vi "SP_OEE_2_test.vi"() -> ()   [LabVIEW 2017] (continued)
                      tunnel: w14784 -> [w15083]
                      tunnel: w14783 -> [w15091]
                      tunnel: w14782 -> [w15081]
                      tunnel: w14781 -> [w15090]
                      tunnel: w14780 -> [w15079]
                      tunnel: w14779 -> [w15089]
                      tunnel: w14778 -> [w15077]
                      tunnel: w14777 -> [w15113]
                      tunnel: w14776 -> [w15112]
                      tunnel: w14775 -> [w15088]
                      tunnel: w14774 -> [w15075]
                      tunnel: [w15113] -> w14772
                      tunnel: [w15112] -> w14771
                      tunnel: [w15106] -> w14770
                      tunnel: [w15099] -> w14769
                      tunnel: [w15098] -> w14768
                      tunnel: [w15097] -> w14767
                      tunnel: [w15096] -> w14766
                      tunnel: [w15095] -> w14765
                      tunnel: [w15094] -> w14764
                      tunnel: [w15093] -> w14763
                      tunnel: [w15092] -> w14762
                      tunnel: [w15091] -> w14761
                      tunnel: [w15090] -> w14760
                      tunnel: [w15089] -> w14759
                      tunnel: [w15088] -> w14758
                      tunnel: [w15073] -> w14757
                      tunnel: w14773 -> [w15073]
                      tunnel: [w15126] -> _
                      tunnel: [w15122] -> _
                      tunnel: w14772 -> [w15123]
                      tunnel: w14771 -> [w15126]
                      tunnel: w14770 -> [w15117]
                      tunnel: w14769 -> [w15124]
                      tunnel: w14768 -> [_]
                      tunnel: w14767 -> [_]
                      tunnel: w14766 -> [w15116]
                      tunnel: w14765 -> [_]
                      tunnel: w14764 -> [_]
                      tunnel: w14763 -> [w15118]
                      tunnel: w14762 -> [_]
                      tunnel: w14761 -> [_]
                      tunnel: w14760 -> [w15114]
                      tunnel: w14759 -> [_]
                      tunnel: w14758 -> [_]
                      tunnel: w14757 -> [w15121]
                      frame #0 {
                        w14861 = "%Y-%m-%d" ("time format string (%c)")
                        n2698 = Decimal String To Number(string=w14847) -> (number=w14848:i32)  [unwired: 2 in, 1 out]
                        n2699 = property on="Table" class="Tbl (strict)"("Visible"=TRUE) -> ()  [unwired: 2 in, 2 out]
                        n2700 = Format Date/Time String(time format string (%c)=w14861, seconds (now)=w14853) -> (date/time string=w14862:string)  [unwired: 1 in]
                        n2701 = Format Date/Time String(time format string (%c)=w14861, seconds (now)=w14852) -> (date/time string=w14860:string)  [unwired: 1 in]
                        n2702 = Format Into String(format string="Where BREAKDOWN_DATE between '%s' and '%s' and  SHIFT_ID = '%d'  ", w14862, w14860, w14848) -> (resulting string=w14859:string)  [unwired: 2 in, 1 out]
                        n2703 = call <vilib>:"DB Tools Select Data.vi"("condition"=w14859, "error in (no error)"=w14868, "columns"=string[] ["BREAKDOWN_DATE"], "table"="STATION_1_LOG_HISTORY", "connection reference"=w14870) -> ("error out"=w14855:errorcluster, "data"=w14858:variant[][], "connection reference out"=w14869:T2)  [unwired: 1 in]
                        n2704 = property on="Table 2" class="Tbl (strict)"("Visible"=FALSE) -> ()  [unwired: 2 in, 2 out]
                        n2705 = xnode "Database Variant To Data"("database variant"=w14858, "error in (no error)"=w14855, "type"=string[][] [] ("Elements Found")) -> ("data"=w14856:string[][], "error out"=w14854:errorcluster)
                        n2706 = Index Array(array=w14856, index (col)=0 ("disabled index (col)")) -> (element=w14864:string[])  [unwired: 1 in]
                        n2707 = call "Search_1d_array_element.vi"("Count in"=string[] [] ("Elements Found"), "BD Date"=w14864, "Elements Found in"=string[] [] ("Elements Found")) -> ("Elements Found out"=w14851:string[])  [unwired: 4 in, 2 out]
                        n2708 = Build Array(w14851) -> (w14874:string[][])
                        n2709 = Transpose 2D Array(2D array=w14874) -> (transposed array=w14873:string[][])
                      }
                      frame #1 {
                        n2710 = disable-structure shown="Enabled" {
                          disable-tunnel: w14936 -> [w14947 w14949]
                          disable-tunnel: [w14946 w14949] -> w14935
                          disable-tunnel: w14934 -> [w14945 w14950]
                          disable-tunnel: [w14944 w14950] -> w14933
                          disable-tunnel: w14931 -> [w14942 _]
                          disable-tunnel: w14930 -> [w14941 _]
                          disable-tunnel: [w14940 _] -> w14929
                          disable-tunnel: [w14939 _] -> w14926
                          disable-tunnel: w14924 -> [w14938 _]
                          disable-tunnel: w14921 -> [w14937 w14948]
                          disable-tunnel: [_ w14948] -> w14920
                          frame Disabled {
                            n2711 = call "Stack_holderwise_total_bd_count_&_duration_2.vi"("Refnum in"=w14947, "BREAKDOWN_STK_HOLD_ID"=1, "condition"=w14938, "Form Date"=w14942, "To Date"=w14941, "error in (no error)"=w14945, "Shift"=w14937) -> ("Refnum out"=w14946:T2, "Count out"=w14940:string[], "appended array"=w14939:dbl[], "error out"=w14944:errorcluster)  [unwired: 5 in]
                          }
                          frame Enabled {
                          }
                        }
                        n2712 = call "NUMERIC TO STRING.vi"("appended array"=w14926) -> ("Array"=w14925:string[])  [unwired: 4 in]
                        n2713 = call "Insert_empty_element_with_zero.vi"("searched date"=w14929, "fixed date"=w14927) -> ("O/P"=w14922:string[])  [unwired: 9 in]
                        n2714 = call "Insert_empty_element_with_zero.vi"("searched date"=w14925, "fixed date"=w14927) -> ("O/P"=w14928:string[])  [unwired: 9 in]
                      }
                      frame #2 {
                        n2715 = disable-structure shown="Enabled" {
                          disable-tunnel: w14966 -> [w14980 w14982]
                          disable-tunnel: [w14979 w14982] -> w14965
                          disable-tunnel: w14964 -> [w14978 w14983]
                          disable-tunnel: [w14977 w14983] -> w14963
                          disable-tunnel: w14962 -> [w14976 _]
                          disable-tunnel: w14961 -> [w14975 _]
                          disable-tunnel: [w14974 _] -> w14960
                          disable-tunnel: [w14973 _] -> w14956
                          disable-tunnel: w14954 -> [w14972 _]
                          disable-tunnel: w14952 -> [w14970 w14981]
                          disable-tunnel: [_ w14981] -> w14951
                          frame Disabled {
                            n2716 = call "Stack_holderwise_total_bd_count_&_duration_2.vi"("Refnum in"=w14978, "BREAKDOWN_STK_HOLD_ID"=2, "condition"=w14972, "Form Date"=w14976, "To Date"=w14975, "error in (no error)"=w14980, "Shift"=w14970) -> ("Refnum out"=w14977:T2, "Count out"=w14974:string[], "appended array"=w14973:dbl[], "error out"=w14979:errorcluster)  [unwired: 5 in]
                          }
                          frame Enabled {
                          }
                        }
                        n2717 = call "Insert_empty_element_with_zero.vi"("searched date"=w14960, "fixed date"=w14957) -> ("O/P"=w14959:string[])  [unwired: 9 in]
                        n2718 = call "NUMERIC TO STRING.vi"("appended array"=w14956) -> ("Array"=w14955:string[])  [unwired: 4 in]
                        n2719 = call "Insert_empty_element_with_zero.vi"("searched date"=w14955, "fixed date"=w14957) -> ("O/P"=w14958:string[])  [unwired: 9 in]
                      }
                      frame #3 {
                        n2720 = call "Stack_holderwise_total_bd_count_&_duration_2.vi"("Refnum in"=w14997, "BREAKDOWN_STK_HOLD_ID"=3, "condition"=w14987, "Form Date"=w14995, "To Date"=w14994, "error in (no error)"=w14999, "Shift"=w14984) -> ("Refnum out"=w14996:T2, "Count out"=w14993:string[], "appended array"=w14989:dbl[], "error out"=w14998:errorcluster)  [unwired: 5 in]
                        n2721 = call "Insert_empty_element_with_zero.vi"("searched date"=w14993, "fixed date"=w14990) -> ("O/P"=w14992:string[])  [unwired: 9 in]
                        n2722 = call "NUMERIC TO STRING.vi"("appended array"=w14989) -> ("Array"=w14988:string[])  [unwired: 4 in]
                        n2723 = call "Insert_empty_element_with_zero.vi"("searched date"=w14988, "fixed date"=w14990) -> ("O/P"=w14991:string[])  [unwired: 9 in]
                      }
                      frame #4 {
                        n2724 = disable-structure shown="Enabled" {
                          disable-tunnel: w15018 -> [w15034 w15037]
                          disable-tunnel: w15017 -> [w15033 w15036]
                          disable-tunnel: [w15032 w15036] -> w15016
                          disable-tunnel: [w15031 w15037] -> w15015
                          disable-tunnel: w15014 -> [w15030 _]
                          disable-tunnel: w15013 -> [w15029 _]
                          disable-tunnel: [w15028 _] -> w15012
                          disable-tunnel: [w15027 _] -> w15008
                          disable-tunnel: w15006 -> [w15026 _]
                          frame Disabled {
                            n2725 = call "Stack_holderwise_total_bd_count_&_duration.vi"("Refnum in"=w15033, "BREAKDOWN_STK_HOLD_ID"=4, "condition"=w15026, "Form Date"=w15030, "To Date"=w15029, "error in (no error)"=w15034) -> ("Refnum out"=w15032:T2, "Count out"=w15028:string[], "appended array"=w15027:dbl[], "error out"=w15031:errorcluster)  [unwired: 6 in]
                          }
                          frame Enabled {
                          }
                        }
                        n2726 = call "Insert_empty_element_with_zero.vi"("searched date"=w15012, "fixed date"=w15009) -> ("O/P"=w15011:string[])  [unwired: 9 in]
                        n2727 = call "NUMERIC TO STRING.vi"("appended array"=w15008) -> ("Array"=w15007:string[])  [unwired: 4 in]
                        n2728 = call "Insert_empty_element_with_zero.vi"("searched date"=w15007, "fixed date"=w15009) -> ("O/P"=w15010:string[])  [unwired: 9 in]
                      }
                      frame #5 {
                        n2729 = disable-structure shown="Enabled" {
                          disable-tunnel: w15051 -> [w15069 w15072]
                          disable-tunnel: [w15068 w15072] -> w15050
                          disable-tunnel: w15049 -> [w15067 w15071]
                          disable-tunnel: [w15066 w15071] -> w15048
                          disable-tunnel: w15047 -> [w15065 _]
                          disable-tunnel: w15046 -> [w15064 _]
                          disable-tunnel: [w15063 _] -> w15045
                          disable-tunnel: [w15062 _] -> w15041
                          disable-tunnel: w15039 -> [w15061 _]
                          frame Disabled {
                            n2730 = call "Stack_holderwise_total_bd_count_&_duration.vi"("Refnum in"=w15067, "BREAKDOWN_STK_HOLD_ID"=5, "condition"=w15061, "Form Date"=w15064, "To Date"=w15065, "error in (no error)"=w15069) -> ("Refnum out"=w15066:T2, "Count out"=w15063:string[], "appended array"=w15062:dbl[], "error out"=w15068:errorcluster)  [unwired: 6 in]
                          }
                          frame Enabled {
                          }
                        }
                        n2731 = call "NUMERIC TO STRING.vi"("appended array"=w15041) -> ("Array"=w15040:string[])  [unwired: 4 in]
                        n2732 = call "Insert_empty_element_with_zero.vi"("searched date"=w15045, "fixed date"=w15043) -> ("O/P"=w15044:string[])  [unwired: 9 in]
                        n2733 = call "Insert_empty_element_with_zero.vi"("searched date"=w15040, "fixed date"=w15043) -> ("O/P"=w15042:string[])  [unwired: 9 in]
                      }
                      frame #6 {
                        n2734 = call "String to numeric.vi"("Array"=w15083) -> ("Array 2"=w15082:dbl[])  [unwired: 4 in]
                        n2735 = call "String to numeric.vi"("Array"=w15081) -> ("Array 2"=w15080:dbl[])  [unwired: 4 in]
                        n2736 = call "String to numeric.vi"("Array"=w15079) -> ("Array 2"=w15078:dbl[])  [unwired: 4 in]
                        n2737 = call "String to numeric.vi"("Array"=w15077) -> ("Array 2"=w15076:dbl[])  [unwired: 4 in]
                        n2738 = call "String to numeric.vi"("Array"=w15075) -> ("Array 2"=w15074:dbl[])  [unwired: 4 in]
                        n2739 = Decimal String To Number(string=w15088) -> (number=w15107:i32[])  [unwired: 2 in, 1 out]
                        n2740 = Decimal String To Number(string=w15089) -> (number=w15108:i32[])  [unwired: 2 in, 1 out]
                        n2741 = Decimal String To Number(string=w15090) -> (number=w15109:i32[])  [unwired: 2 in, 1 out]
                        n2742 = Decimal String To Number(string=w15091) -> (number=w15110:i32[])  [unwired: 2 in, 1 out]
                        n2743 = Decimal String To Number(string=w15092) -> (number=w15105:i32[])  [unwired: 2 in, 1 out]
                        n2744 = Compound Arithmetic op=ADD(w15082, w15080, w15078, w15076, w15074) -> (w15085:dbl[])
                        n2745 = Build Array(w15083) -> (w15104:string[][])
                        n2746 = Build Array(w15081) -> (w15103:string[][])
                        n2747 = Build Array(w15079) -> (w15102:string[][])
                        n2748 = Build Array(w15077) -> (w15101:string[][])
                        n2749 = Build Array(w15075) -> (w15100:string[][])
                        n2750 = Number To Fractional String(number=w15085, precision (6)=i16 2) -> (F-format string=w15084:string[])  [unwired: 2 in]
                        n2751 = Compound Arithmetic op=ADD(w15107, w15108, w15109, w15110, w15105) -> (w15111:i32[])
                        n2752 = Transpose 2D Array(2D array=w15104) -> (transposed array=w15098:string[][])
                        n2753 = Transpose 2D Array(2D array=w15103) -> (transposed array=w15097:string[][])
                        n2754 = Transpose 2D Array(2D array=w15102) -> (transposed array=w15096:string[][])
                        n2755 = Transpose 2D Array(2D array=w15101) -> (transposed array=w15095:string[][])
                        n2756 = Transpose 2D Array(2D array=w15100) -> (transposed array=w15094:string[][])
                        n2757 = Number To Decimal String(number=w15111) -> (decimal integer string=w15106:string[])  [unwired: 1 in]
                        n2758 = Build Array(w15084) -> (w15087:string[][])
                        n2759 = Transpose 2D Array(2D array=w15087) -> (transposed array=w15093:string[][])
                      }
                      frame #7 {
                        w15115 = string[] [""]
                        n2760 = Insert Into Array(array=w15124, index (col)=1 ("disabled index (col)"), new element #1=w15115, new element #2=w15115, new element #3=w15115, new element #4=w15115, new element #5=w15114, new element #6=w15116, new element #7=w15115, new element #8=w15115, new element #9=w15115, new element #10=w15115, new element #11=w15117, new element #12=w15118) -> (w15120:string[][])  [unwired: 1 in]
                        n2761 = call "flot graph for month n year.vi"("BD Date"=w15121, "error in (no error)"=w15123, "Count total"=w15117) -> ("error out"=w15122:errorcluster, "Run-Time Status"=w15119:cluster{"Array 2":timestamp[], dbl[]})  [unwired: 7 in]
                        n2762 = local write "Run-Time Status"(w15119) -> ()
                        n2763 = local write "Table"(w15120) -> ()
                      }
                    }
                  }
                  frame "all" {
                  }
                }
              }
              frame "Quality" {
                n2764 = local read "Shift"() -> (w15127:string)
                n2765 = case shown="\"3\"" w15127 {
                  selector: w15127 -> [_ w15501 w15885 w16269 _]
                  tunnel: w15132 -> [w15137 w15506 w15890 w16274 _]
                  tunnel: w15131 -> [w15136 w15505 w15889 w16273 _]
                  tunnel: w15130 -> [w15135 w15504 w15888 w16272 _]
                  tunnel: w15129 -> [w15134 w15503 w15887 w16271 _]
                  tunnel: w15128 -> [w15133 w15502 w15886 w16270 _]
                  frame "ALL", Default {
                    n2766 = flat-sequence {
                      tunnel: w15137 -> [w15249]
                      tunnel: w15136 -> [w15247]
                      tunnel: [w15233] -> w15227
                      tunnel: [w15248] -> w15226
                      tunnel: w15135 -> [_]
                      tunnel: [w15252] -> w15225
                      tunnel: [w15232] -> w15224
                      tunnel: [w15231] -> w15223
                      tunnel: [w15229] -> w15222
                      tunnel: w15134 -> [w15232]
                      tunnel: w15133 -> [w15231]
                      tunnel: ["Where BREAKDOWN_DATE between '%s'and '%s' and BREAKDOWN_STK_HOLD_ID ='%d'  "] -> w15221
                      tunnel: [w15229] -> w15220
                      tunnel: w15227 -> [w15311]
                      tunnel: w15226 -> [w15313]
                      tunnel: w15225 -> [w15309]
                      tunnel: w15224 -> [w15308]
                      tunnel: w15223 -> [w15307]
                      tunnel: [w15310] -> w15219
                      tunnel: [w15312] -> w15218
                      tunnel: [w15309] -> w15217
                      tunnel: [w15299] -> w15216
                      tunnel: [w15305] -> w15215
                      tunnel: [w15308] -> w15214
                      tunnel: [w15307] -> w15213
                      tunnel: w15222 -> [w15304]
                      tunnel: [w15304] -> w15212
                      tunnel: w15221 -> [w15301]
                      tunnel: [w15301] -> w15211
                      tunnel: [w15300] -> w15210
                      tunnel: w15220 -> [w15300]
                      tunnel: w15219 -> [w15339]
                      tunnel: w15218 -> [w15337]
                      tunnel: w15217 -> [w15342]
                      tunnel: w15216 -> [w15341]
                      tunnel: w15215 -> [w15340]
                      tunnel: w15214 -> [w15335]
                      tunnel: w15213 -> [w15334]
                      tunnel: [w15342] -> w15209
                      tunnel: [w15341] -> w15208
                      tunnel: [w15340] -> w15207
                      tunnel: [w15338] -> w15206
                      tunnel: [w15332] -> w15205
                      tunnel: [w15331] -> w15204
                      tunnel: [w15336] -> w15203
                      tunnel: [w15335] -> w15202
                      tunnel: [w15334] -> w15201
                      tunnel: w15212 -> [w15330]
                      tunnel: [w15330] -> w15200
                      tunnel: w15211 -> [w15327]
                      tunnel: [w15327] -> w15199
                      tunnel: [w15326] -> w15198
                      tunnel: w15210 -> [w15326]
                      tunnel: w15209 -> [w15373]
                      tunnel: w15208 -> [w15372]
                      tunnel: w15207 -> [w15371]
                      tunnel: w15206 -> [w15368]
                      tunnel: w15205 -> [w15370]
                      tunnel: w15204 -> [w15369]
                      tunnel: w15203 -> [w15366]
                      tunnel: w15202 -> [w15364]
                      tunnel: w15201 -> [w15363]
                      tunnel: [w15373] -> w15197
                      tunnel: [w15372] -> w15196
                      tunnel: [w15371] -> w15195
                      tunnel: [w15370] -> w15194
                      tunnel: [w15369] -> w15193
                      tunnel: [w15367] -> w15192
                      tunnel: [w15361] -> w15191
                      tunnel: [w15360] -> w15190
                      tunnel: [w15365] -> w15189
                      tunnel: [w15364] -> w15188
                      tunnel: [w15363] -> w15187
                      tunnel: w15200 -> [w15359]
                      tunnel: [w15359] -> w15186
                      tunnel: w15199 -> [w15356]
                      tunnel: [w15356] -> w15185
                      tunnel: [w15355] -> w15184
                      tunnel: w15198 -> [w15355]
                      tunnel: w15197 -> [w15407]
                      tunnel: w15196 -> [w15406]
                      tunnel: w15195 -> [w15405]
                      tunnel: w15194 -> [w15404]
                      tunnel: w15193 -> [w15403]
                      tunnel: w15192 -> [w15400]
                      tunnel: w15191 -> [w15402]
                      tunnel: w15190 -> [w15401]
                      tunnel: w15189 -> [w15399]
                      tunnel: w15188 -> [w15396]
                      tunnel: w15187 -> [w15395]
                      tunnel: [w15407] -> w15183
                      tunnel: [w15406] -> w15182
                      tunnel: [w15405] -> w15181
                      tunnel: [w15404] -> w15180
                      tunnel: [w15403] -> w15179
                      tunnel: [w15402] -> w15178
                      tunnel: [w15401] -> w15177
                      tunnel: [w15398] -> w15176
                      tunnel: [w15397] -> w15175
                      tunnel: [w15393] -> w15174
                      tunnel: [w15392] -> w15173
                      tunnel: [w15396] -> w15172
                      tunnel: [w15395] -> w15171
                      tunnel: w15186 -> [w15391]
                      tunnel: [w15391] -> w15170
                      tunnel: w15185 -> [w15388]
                      tunnel: [w15388] -> w15169
                      tunnel: [w15387] -> w15168
                      tunnel: w15184 -> [w15387]
                      tunnel: w15183 -> [w15430]
                      tunnel: w15182 -> [w15429]
                      tunnel: w15181 -> [w15428]
                      tunnel: w15180 -> [w15427]
                      tunnel: w15179 -> [w15426]
                      tunnel: w15178 -> [w15425]
                      tunnel: w15177 -> [w15424]
                      tunnel: w15176 -> [w15419]
                      tunnel: w15175 -> [w15421]
                      tunnel: w15174 -> [w15423]
                      tunnel: w15173 -> [w15422]
                      tunnel: w15172 -> [w15416]
                      tunnel: w15171 -> [w15417]
                      tunnel: [w15430] -> w15167
                      tunnel: [w15429] -> w15166
                      tunnel: [w15428] -> w15165
                      tunnel: [w15427] -> w15164
                      tunnel: [w15426] -> w15163
                      tunnel: [w15425] -> w15162
                      tunnel: [w15424] -> w15161
                      tunnel: [w15423] -> w15160
                      tunnel: [w15422] -> w15159
                      tunnel: [w15420] -> w15158
                      tunnel: [w15418] -> w15157
                      tunnel: [w15414] -> w15156
                      tunnel: [w15412] -> w15155
                      tunnel: w15170 -> [w15413]
                      tunnel: w15169 -> [w15409]
                      tunnel: [w15408] -> w15154
                      tunnel: w15168 -> [w15408]
                      tunnel: w15167 -> [w15469]
                      tunnel: w15166 -> [w15462]
                      tunnel: w15165 -> [w15453]
                      tunnel: w15164 -> [w15461]
                      tunnel: w15163 -> [w15451]
                      tunnel: w15162 -> [w15460]
                      tunnel: w15161 -> [w15449]
                      tunnel: w15160 -> [w15459]
                      tunnel: w15159 -> [w15447]
                      tunnel: w15158 -> [w15483]
                      tunnel: w15157 -> [w15482]
                      tunnel: w15156 -> [w15458]
                      tunnel: w15155 -> [w15445]
                      tunnel: [w15483] -> w15153
                      tunnel: [w15482] -> w15152
                      tunnel: [w15476] -> w15151
                      tunnel: [w15469] -> w15150
                      tunnel: [w15468] -> w15149
                      tunnel: [w15467] -> w15148
                      tunnel: [w15466] -> w15147
                      tunnel: [w15465] -> w15146
                      tunnel: [w15464] -> w15145
                      tunnel: [w15463] -> w15144
                      tunnel: [w15462] -> w15143
                      tunnel: [w15461] -> w15142
                      tunnel: [w15460] -> w15141
                      tunnel: [w15459] -> w15140
                      tunnel: [w15458] -> w15139
                      tunnel: [w15443] -> w15138
                      tunnel: w15154 -> [w15443]
                      tunnel: [w15496] -> _
                      tunnel: [w15492] -> _
                      tunnel: w15153 -> [w15493]
                      tunnel: w15152 -> [w15496]
                      tunnel: w15151 -> [w15487]
                      tunnel: w15150 -> [w15494]
                      tunnel: w15149 -> [_]
                      tunnel: w15148 -> [_]
                      tunnel: w15147 -> [_]
                      tunnel: w15146 -> [w15484]
                      tunnel: w15145 -> [_]
                      tunnel: w15144 -> [w15488]
                      tunnel: w15143 -> [_]
                      tunnel: w15142 -> [_]
                      tunnel: w15141 -> [_]
                      tunnel: w15140 -> [w15485]
                      tunnel: w15139 -> [_]
                      tunnel: w15138 -> [w15491]
                      frame #0 {
                        w15240 = "%Y-%m-%d" ("time format string (%c)")
                        n2767 = property on="Table" class="Tbl (strict)"("Visible"=TRUE) -> ()  [unwired: 2 in, 2 out]
                        n2768 = Format Date/Time String(time format string (%c)=w15240, seconds (now)=w15232) -> (date/time string=w15241:string)  [unwired: 1 in]
                        n2769 = Format Date/Time String(time format string (%c)=w15240, seconds (now)=w15231) -> (date/time string=w15239:string)  [unwired: 1 in]
                        n2770 = Format Into String(format string="Where BREAKDOWN_DATE between '%s' and '%s' ", w15241, w15239) -> (resulting string=w15238:string)  [unwired: 2 in, 1 out]
                        n2771 = call <vilib>:"DB Tools Select Data.vi"("condition"=w15238, "error in (no error)"=w15247, "columns"=string[] ["BREAKDOWN_DATE"], "table"="STATION_1_LOG_HISTORY", "connection reference"=w15249) -> ("error out"=w15234:errorcluster, "data"=w15237:variant[][], "connection reference out"=w15248:T2)  [unwired: 1 in]
                        n2772 = property on="Table 2" class="Tbl (strict)"("Visible"=FALSE) -> ()  [unwired: 2 in, 2 out]
                        n2773 = xnode "Database Variant To Data"("database variant"=w15237, "error in (no error)"=w15234, "type"=string[][] [] ("Elements Found")) -> ("data"=w15235:string[][], "error out"=w15233:errorcluster)
                        n2774 = Index Array(array=w15235, index (col)=0 ("disabled index (col)")) -> (element=w15243:string[])  [unwired: 1 in]
                        n2775 = call "Search_1d_array_element.vi"("Count in"=string[] [] ("Elements Found"), "BD Date"=w15243, "Elements Found in"=string[] [] ("Elements Found")) -> ("Elements Found out"=w15229:string[])  [unwired: 4 in, 2 out]
                        n2776 = Build Array(w15229) -> (w15253:string[][])
                        n2777 = Transpose 2D Array(2D array=w15253) -> (transposed array=w15252:string[][])
                      }
                      frame #1 {
                        n2778 = disable-structure shown="Enabled" {
                          disable-tunnel: w15313 -> [w15323 w15324]
                          disable-tunnel: [w15322 w15324] -> w15312
                          disable-tunnel: w15311 -> [w15321 w15325]
                          disable-tunnel: [w15320 w15325] -> w15310
                          disable-tunnel: w15308 -> [w15318 _]
                          disable-tunnel: w15307 -> [w15317 _]
                          disable-tunnel: [w15316 _] -> w15306
                          disable-tunnel: [w15315 _] -> w15303
                          disable-tunnel: w15301 -> [w15314 _]
                          frame Disabled {
                            n2779 = call "Stack_holderwise_total_bd_count_&_duration.vi"("Refnum in"=w15323, "BREAKDOWN_STK_HOLD_ID"=1, "condition"=w15314, "Form Date"=w15318, "To Date"=w15317, "error in (no error)"=w15321) -> ("Refnum out"=w15322:T2, "Count out"=w15316:string[], "appended array"=w15315:dbl[], "error out"=w15320:errorcluster)  [unwired: 6 in]
                          }
                          frame Enabled {
                          }
                        }
                        n2780 = call "NUMERIC TO STRING.vi"("appended array"=w15303) -> ("Array"=w15302:string[])  [unwired: 4 in]
                        n2781 = call "Insert_empty_element_with_zero.vi"("searched date"=w15306, "fixed date"=w15304) -> ("O/P"=w15299:string[])  [unwired: 9 in]
                        n2782 = call "Insert_empty_element_with_zero.vi"("searched date"=w15302, "fixed date"=w15304) -> ("O/P"=w15305:string[])  [unwired: 9 in]
                      }
                      frame #2 {
                        n2783 = disable-structure shown="Enabled" {
                          disable-tunnel: w15339 -> [w15352 w15354]
                          disable-tunnel: [w15351 w15354] -> w15338
                          disable-tunnel: w15337 -> [w15350 w15353]
                          disable-tunnel: [w15349 w15353] -> w15336
                          disable-tunnel: w15335 -> [w15348 _]
                          disable-tunnel: w15334 -> [w15347 _]
                          disable-tunnel: [w15346 _] -> w15333
                          disable-tunnel: [w15345 _] -> w15329
                          disable-tunnel: w15327 -> [w15344 _]
                          frame Disabled {
                            n2784 = call "Stack_holderwise_total_bd_count_&_duration.vi"("Refnum in"=w15350, "BREAKDOWN_STK_HOLD_ID"=2, "condition"=w15344, "Form Date"=w15348, "To Date"=w15347, "error in (no error)"=w15352) -> ("Refnum out"=w15349:T2, "Count out"=w15346:string[], "appended array"=w15345:dbl[], "error out"=w15351:errorcluster)  [unwired: 6 in]
                          }
                          frame Enabled {
                          }
                        }
                        n2785 = call "Insert_empty_element_with_zero.vi"("searched date"=w15333, "fixed date"=w15330) -> ("O/P"=w15332:string[])  [unwired: 9 in]
                        n2786 = call "NUMERIC TO STRING.vi"("appended array"=w15329) -> ("Array"=w15328:string[])  [unwired: 4 in]
                        n2787 = call "Insert_empty_element_with_zero.vi"("searched date"=w15328, "fixed date"=w15330) -> ("O/P"=w15331:string[])  [unwired: 9 in]
                      }
                      frame #3 {
                        n2788 = disable-structure shown="Enabled" {
                          disable-tunnel: w15368 -> [w15383 w15385]
                          disable-tunnel: [w15382 w15385] -> w15367
                          disable-tunnel: w15366 -> [w15381 w15384]
                          disable-tunnel: [w15380 w15384] -> w15365
                          disable-tunnel: w15364 -> [w15379 _]
                          disable-tunnel: w15363 -> [w15378 _]
                          disable-tunnel: [w15377 _] -> w15362
                          disable-tunnel: [w15376 _] -> w15358
                          disable-tunnel: w15356 -> [w15375 _]
                          frame Disabled {
                            n2789 = call "Stack_holderwise_total_bd_count_&_duration.vi"("Refnum in"=w15381, "BREAKDOWN_STK_HOLD_ID"=3, "condition"=w15375, "Form Date"=w15379, "To Date"=w15378, "error in (no error)"=w15383) -> ("Refnum out"=w15380:T2, "Count out"=w15377:string[], "appended array"=w15376:dbl[], "error out"=w15382:errorcluster)  [unwired: 6 in]
                          }
                          frame Enabled {
                          }
                        }
                        n2790 = call "Insert_empty_element_with_zero.vi"("searched date"=w15362, "fixed date"=w15359) -> ("O/P"=w15361:string[])  [unwired: 9 in]
                        n2791 = call "NUMERIC TO STRING.vi"("appended array"=w15358) -> ("Array"=w15357:string[])  [unwired: 4 in]
                        n2792 = call "Insert_empty_element_with_zero.vi"("searched date"=w15357, "fixed date"=w15359) -> ("O/P"=w15360:string[])  [unwired: 9 in]
                      }
                      frame #4 {
                        n2793 = call "Stack_holderwise_total_bd_count_&_duration.vi"("Refnum in"=w15399, "BREAKDOWN_STK_HOLD_ID"=4, "condition"=w15388, "Form Date"=w15396, "To Date"=w15395, "error in (no error)"=w15400) -> ("Refnum out"=w15398:T2, "Count out"=w15394:string[], "appended array"=w15390:dbl[], "error out"=w15397:errorcluster)  [unwired: 6 in]
                        n2794 = call "Insert_empty_element_with_zero.vi"("searched date"=w15394, "fixed date"=w15391) -> ("O/P"=w15393:string[])  [unwired: 9 in]
                        n2795 = call "NUMERIC TO STRING.vi"("appended array"=w15390) -> ("Array"=w15389:string[])  [unwired: 4 in]
                        n2796 = call "Insert_empty_element_with_zero.vi"("searched date"=w15389, "fixed date"=w15391) -> ("O/P"=w15392:string[])  [unwired: 9 in]
                      }
                      frame #5 {
                        n2797 = disable-structure shown="Enabled" {
                          disable-tunnel: w15421 -> [w15439 w15442]
                          disable-tunnel: [w15438 w15442] -> w15420
                          disable-tunnel: w15419 -> [w15437 w15441]
                          disable-tunnel: [w15436 w15441] -> w15418
                          disable-tunnel: w15417 -> [w15435 _]
                          disable-tunnel: w15416 -> [w15434 _]
                          disable-tunnel: [w15433 _] -> w15415
                          disable-tunnel: [w15432 _] -> w15411
                          disable-tunnel: w15409 -> [w15431 _]
                          frame Disabled {
                            n2798 = call "Stack_holderwise_total_bd_count_&_duration.vi"("Refnum in"=w15437, "BREAKDOWN_STK_HOLD_ID"=5, "condition"=w15431, "Form Date"=w15434, "To Date"=w15435, "error in (no error)"=w15439) -> ("Refnum out"=w15436:T2, "Count out"=w15433:string[], "appended array"=w15432:dbl[], "error out"=w15438:errorcluster)  [unwired: 6 in]
                          }
                          frame Enabled {
                          }
                        }
                        n2799 = call "NUMERIC TO STRING.vi"("appended array"=w15411) -> ("Array"=w15410:string[])  [unwired: 4 in]
                        n2800 = call "Insert_empty_element_with_zero.vi"("searched date"=w15415, "fixed date"=w15413) -> ("O/P"=w15414:string[])  [unwired: 9 in]
                        n2801 = call "Insert_empty_element_with_zero.vi"("searched date"=w15410, "fixed date"=w15413) -> ("O/P"=w15412:string[])  [unwired: 9 in]
                      }
                      frame #6 {
                        n2802 = call "String to numeric.vi"("Array"=w15453) -> ("Array 2"=w15452:dbl[])  [unwired: 4 in]
                        n2803 = call "String to numeric.vi"("Array"=w15451) -> ("Array 2"=w15450:dbl[])  [unwired: 4 in]
                        n2804 = call "String to numeric.vi"("Array"=w15449) -> ("Array 2"=w15448:dbl[])  [unwired: 4 in]
                        n2805 = call "String to numeric.vi"("Array"=w15447) -> ("Array 2"=w15446:dbl[])  [unwired: 4 in]
                        n2806 = call "String to numeric.vi"("Array"=w15445) -> ("Array 2"=w15444:dbl[])  [unwired: 4 in]
                        n2807 = Decimal String To Number(string=w15458) -> (number=w15477:i32[])  [unwired: 2 in, 1 out]
                        n2808 = Decimal String To Number(string=w15459) -> (number=w15478:i32[])  [unwired: 2 in, 1 out]
                        n2809 = Decimal String To Number(string=w15460) -> (number=w15479:i32[])  [unwired: 2 in, 1 out]
                        n2810 = Decimal String To Number(string=w15461) -> (number=w15480:i32[])  [unwired: 2 in, 1 out]
                        n2811 = Decimal String To Number(string=w15462) -> (number=w15475:i32[])  [unwired: 2 in, 1 out]
                        n2812 = Compound Arithmetic op=ADD(w15452, w15450, w15448, w15446, w15444) -> (w15455:dbl[])
                        n2813 = Build Array(w15453) -> (w15474:string[][])
                        n2814 = Build Array(w15451) -> (w15473:string[][])
                        n2815 = Build Array(w15449) -> (w15472:string[][])
                        n2816 = Build Array(w15447) -> (w15471:string[][])
                        n2817 = Build Array(w15445) -> (w15470:string[][])
                        n2818 = Number To Fractional String(number=w15455, precision (6)=i16 2) -> (F-format string=w15454:string[])  [unwired: 2 in]
                        n2819 = Compound Arithmetic op=ADD(w15477, w15478, w15479, w15480, w15475) -> (w15481:i32[])
                        n2820 = Transpose 2D Array(2D array=w15474) -> (transposed array=w15468:string[][])
                        n2821 = Transpose 2D Array(2D array=w15473) -> (transposed array=w15467:string[][])
                        n2822 = Transpose 2D Array(2D array=w15472) -> (transposed array=w15466:string[][])
                        n2823 = Transpose 2D Array(2D array=w15471) -> (transposed array=w15465:string[][])
                        n2824 = Transpose 2D Array(2D array=w15470) -> (transposed array=w15464:string[][])
                        n2825 = Number To Decimal String(number=w15481) -> (decimal integer string=w15476:string[])  [unwired: 1 in]
                        n2826 = Build Array(w15454) -> (w15457:string[][])
                        n2827 = Transpose 2D Array(2D array=w15457) -> (transposed array=w15463:string[][])
                      }
                      frame #7 {
                        w15486 = string[] [""]
                        n2828 = Insert Into Array(array=w15494, index (col)=1 ("disabled index (col)"), new element #1=w15486, new element #2=w15486, new element #3=w15486, new element #4=w15486, new element #5=w15486, new element #6=w15486, new element #7=w15485, new element #8=w15484, new element #9=w15486, new element #10=w15486, new element #11=w15487, new element #12=w15488) -> (w15490:string[][])  [unwired: 1 in]
                        n2829 = call "flot graph for month n year.vi"("BD Date"=w15491, "error in (no error)"=w15493, "Count total"=w15487) -> ("error out"=w15492:errorcluster, "Run-Time Status"=w15489:cluster{"Array 2":timestamp[], dbl[]})  [unwired: 7 in]
                        n2830 = local write "Run-Time Status"(w15489) -> ()
                        n2831 = local write "Table"(w15490) -> ()
                      }
                    }
                  }
                  frame "1" {
                    n2832 = flat-sequence {
                      tunnel: w15506 -> [w15620]
                      tunnel: w15505 -> [w15618]
                      tunnel: [w15604] -> w15596
                      tunnel: [w15619] -> w15595
                      tunnel: w15504 -> [_]
                      tunnel: [w15623] -> w15594
                      tunnel: [w15603] -> w15593
                      tunnel: [w15602] -> w15592
                      tunnel: [w15601] -> w15591
                      tunnel: w15503 -> [w15603]
                      tunnel: w15502 -> [w15602]
                      tunnel: ["Where BREAKDOWN_DATE between '%s'and '%s' and BREAKDOWN_STK_HOLD_ID ='%d' and  SHIFT_ID = '%d' "] -> w15590
                      tunnel: [w15601] -> w15589
                      tunnel: w15501 -> [w15597]
                      tunnel: [w15597] -> w15500
                      tunnel: w15596 -> [w15684]
                      tunnel: w15595 -> [w15686]
                      tunnel: w15594 -> [w15682]
                      tunnel: w15593 -> [w15681]
                      tunnel: w15592 -> [w15680]
                      tunnel: [w15683] -> w15588
                      tunnel: [w15685] -> w15587
                      tunnel: [w15682] -> w15586
                      tunnel: [w15672] -> w15585
                      tunnel: [w15678] -> w15584
                      tunnel: [w15681] -> w15583
                      tunnel: [w15680] -> w15582
                      tunnel: w15591 -> [w15677]
                      tunnel: [w15677] -> w15581
                      tunnel: w15590 -> [w15674]
                      tunnel: [w15674] -> w15580
                      tunnel: [w15673] -> w15579
                      tunnel: w15589 -> [w15673]
                      tunnel: w15500 -> [w15671]
                      tunnel: [w15670] -> w15499
                      tunnel: w15588 -> [w15716]
                      tunnel: w15587 -> [w15714]
                      tunnel: w15586 -> [w15719]
                      tunnel: w15585 -> [w15718]
                      tunnel: w15584 -> [w15717]
                      tunnel: w15583 -> [w15712]
                      tunnel: w15582 -> [w15711]
                      tunnel: [w15719] -> w15578
                      tunnel: [w15718] -> w15577
                      tunnel: [w15717] -> w15576
                      tunnel: [w15715] -> w15575
                      tunnel: [w15709] -> w15574
                      tunnel: [w15708] -> w15573
                      tunnel: [w15713] -> w15572
                      tunnel: [w15712] -> w15571
                      tunnel: [w15711] -> w15570
                      tunnel: w15581 -> [w15707]
                      tunnel: [w15707] -> w15569
                      tunnel: w15580 -> [w15704]
                      tunnel: [w15704] -> w15568
                      tunnel: [w15703] -> w15567
                      tunnel: w15579 -> [w15703]
                      tunnel: w15499 -> [w15702]
                      tunnel: [w15701] -> w15498
                      tunnel: w15578 -> [w15754]
                      tunnel: w15577 -> [w15753]
                      tunnel: w15576 -> [w15752]
                      tunnel: w15575 -> [w15749]
                      tunnel: w15574 -> [w15751]
                      tunnel: w15573 -> [w15750]
                      tunnel: w15572 -> [w15747]
                      tunnel: w15571 -> [w15745]
                      tunnel: w15570 -> [w15744]
                      tunnel: [w15754] -> w15566
                      tunnel: [w15753] -> w15565
                      tunnel: [w15752] -> w15564
                      tunnel: [w15751] -> w15563
                      tunnel: [w15750] -> w15562
                      tunnel: [w15748] -> w15561
                      tunnel: [w15742] -> w15560
                      tunnel: [w15741] -> w15559
                      tunnel: [w15746] -> w15558
                      tunnel: [w15745] -> w15557
                      tunnel: [w15744] -> w15556
                      tunnel: w15569 -> [w15740]
                      tunnel: [w15740] -> w15555
                      tunnel: w15568 -> [w15737]
                      tunnel: [w15737] -> w15554
                      tunnel: [w15736] -> w15553
                      tunnel: w15567 -> [w15736]
                      tunnel: w15498 -> [w15735]
                      tunnel: [w15734] -> w15497
                      tunnel: w15566 -> [w15791]
                      tunnel: w15565 -> [w15790]
                      tunnel: w15564 -> [w15789]
                      tunnel: w15563 -> [w15788]
                      tunnel: w15562 -> [w15787]
                      tunnel: w15561 -> [w15784]
                      tunnel: w15560 -> [w15786]
                      tunnel: w15559 -> [w15785]
                      tunnel: w15558 -> [w15783]
                      tunnel: w15557 -> [w15780]
                      tunnel: w15556 -> [w15779]
                      tunnel: [w15791] -> w15552
                      tunnel: [w15790] -> w15551
                      tunnel: [w15789] -> w15550
                      tunnel: [w15788] -> w15549
                      tunnel: [w15787] -> w15548
                      tunnel: [w15786] -> w15547
                      tunnel: [w15785] -> w15546
                      tunnel: [w15782] -> w15545
                      tunnel: [w15781] -> w15544
                      tunnel: [w15777] -> w15543
                      tunnel: [w15776] -> w15542
                      tunnel: [w15780] -> w15541
                      tunnel: [w15779] -> w15540
                      tunnel: w15555 -> [w15775]
                      tunnel: [w15775] -> w15539
                      tunnel: w15554 -> [w15772]
                      tunnel: [w15772] -> w15538
                      tunnel: [w15771] -> w15537
                      tunnel: w15553 -> [w15771]
                      tunnel: w15497 -> [w15769]
                      tunnel: w15552 -> [w15814]
                      tunnel: w15551 -> [w15813]
                      tunnel: w15550 -> [w15812]
                      tunnel: w15549 -> [w15811]
                      tunnel: w15548 -> [w15810]
                      tunnel: w15547 -> [w15809]
                      tunnel: w15546 -> [w15808]
                      tunnel: w15545 -> [w15803]
                      tunnel: w15544 -> [w15805]
                      tunnel: w15543 -> [w15807]
                      tunnel: w15542 -> [w15806]
                      tunnel: w15541 -> [w15800]
                      tunnel: w15540 -> [w15801]
                      tunnel: [w15814] -> w15536
                      tunnel: [w15813] -> w15535
                      tunnel: [w15812] -> w15534
                      tunnel: [w15811] -> w15533
                      tunnel: [w15810] -> w15532
                      tunnel: [w15809] -> w15531
                      tunnel: [w15808] -> w15530
                      tunnel: [w15807] -> w15529
                      tunnel: [w15806] -> w15528
                      tunnel: [w15804] -> w15527
                      tunnel: [w15802] -> w15526
                      tunnel: [w15798] -> w15525
                      tunnel: [w15796] -> w15524
                      tunnel: w15539 -> [w15797]
                      tunnel: w15538 -> [w15793]
                      tunnel: [w15792] -> w15523
                      tunnel: w15537 -> [w15792]
                      tunnel: w15536 -> [w15853]
                      tunnel: w15535 -> [w15846]
                      tunnel: w15534 -> [w15837]
                      tunnel: w15533 -> [w15845]
                      tunnel: w15532 -> [w15835]
                      tunnel: w15531 -> [w15844]
                      tunnel: w15530 -> [w15833]
                      tunnel: w15529 -> [w15843]
                      tunnel: w15528 -> [w15831]
                      tunnel: w15527 -> [w15867]
                      tunnel: w15526 -> [w15866]
                      tunnel: w15525 -> [w15842]
                      tunnel: w15524 -> [w15829]
                      tunnel: [w15867] -> w15522
                      tunnel: [w15866] -> w15521
                      tunnel: [w15860] -> w15520
                      tunnel: [w15853] -> w15519
                      tunnel: [w15852] -> w15518
                      tunnel: [w15851] -> w15517
                      tunnel: [w15850] -> w15516
                      tunnel: [w15849] -> w15515
                      tunnel: [w15848] -> w15514
                      tunnel: [w15847] -> w15513
                      tunnel: [w15846] -> w15512
                      tunnel: [w15845] -> w15511
                      tunnel: [w15844] -> w15510
                      tunnel: [w15843] -> w15509
                      tunnel: [w15842] -> w15508
                      tunnel: [w15827] -> w15507
                      tunnel: w15523 -> [w15827]
                      tunnel: [w15880] -> _
                      tunnel: [w15876] -> _
                      tunnel: w15522 -> [w15877]
                      tunnel: w15521 -> [w15880]
                      tunnel: w15520 -> [w15871]
                      tunnel: w15519 -> [w15878]
                      tunnel: w15518 -> [_]
                      tunnel: w15517 -> [_]
                      tunnel: w15516 -> [_]
                      tunnel: w15515 -> [w15868]
                      tunnel: w15514 -> [_]
                      tunnel: w15513 -> [w15872]
                      tunnel: w15512 -> [_]
                      tunnel: w15511 -> [_]
                      tunnel: w15510 -> [_]
                      tunnel: w15509 -> [w15869]
                      tunnel: w15508 -> [_]
                      tunnel: w15507 -> [w15875]
                      frame #0 {
                        w15611 = "%Y-%m-%d" ("time format string (%c)")
                        n2833 = Decimal String To Number(string=w15597) -> (number=w15598:i32)  [unwired: 2 in, 1 out]
                        n2834 = property on="Table" class="Tbl (strict)"("Visible"=TRUE) -> ()  [unwired: 2 in, 2 out]
                        n2835 = Format Date/Time String(time format string (%c)=w15611, seconds (now)=w15603) -> (date/time string=w15612:string)  [unwired: 1 in]
                        n2836 = Format Date/Time String(time format string (%c)=w15611, seconds (now)=w15602) -> (date/time string=w15610:string)  [unwired: 1 in]
                        n2837 = Format Into String(format string="Where BREAKDOWN_DATE between '%s' and '%s' and  SHIFT_ID = '%d'  ", w15612, w15610, w15598) -> (resulting string=w15609:string)  [unwired: 2 in, 1 out]
                        n2838 = call <vilib>:"DB Tools Select Data.vi"("condition"=w15609, "error in (no error)"=w15618, "columns"=string[] ["BREAKDOWN_DATE"], "table"="STATION_1_LOG_HISTORY", "connection reference"=w15620) -> ("error out"=w15605:errorcluster, "data"=w15608:variant[][], "connection reference out"=w15619:T2)  [unwired: 1 in]
                        n2839 = property on="Table 2" class="Tbl (strict)"("Visible"=FALSE) -> ()  [unwired: 2 in, 2 out]
                        n2840 = xnode "Database Variant To Data"("database variant"=w15608, "error in (no error)"=w15605, "type"=string[][] [] ("Elements Found")) -> ("data"=w15606:string[][], "error out"=w15604:errorcluster)
                        n2841 = Index Array(array=w15606, index (col)=0 ("disabled index (col)")) -> (element=w15614:string[])  [unwired: 1 in]
                        n2842 = call "Search_1d_array_element.vi"("Count in"=string[] [] ("Elements Found"), "BD Date"=w15614, "Elements Found in"=string[] [] ("Elements Found")) -> ("Elements Found out"=w15601:string[])  [unwired: 4 in, 2 out]
                        n2843 = Build Array(w15601) -> (w15624:string[][])
                        n2844 = Transpose 2D Array(2D array=w15624) -> (transposed array=w15623:string[][])
                      }
                      frame #1 {
                        n2845 = disable-structure shown="Enabled" {
                          disable-tunnel: w15686 -> [w15697 w15699]
                          disable-tunnel: [w15696 w15699] -> w15685
                          disable-tunnel: w15684 -> [w15695 w15700]
                          disable-tunnel: [w15694 w15700] -> w15683
                          disable-tunnel: w15681 -> [w15692 _]
                          disable-tunnel: w15680 -> [w15691 _]
                          disable-tunnel: [w15690 _] -> w15679
                          disable-tunnel: [w15689 _] -> w15676
                          disable-tunnel: w15674 -> [w15688 _]
                          disable-tunnel: w15671 -> [w15687 w15698]
                          disable-tunnel: [_ w15698] -> w15670
                          frame Disabled {
                            n2846 = call "Stack_holderwise_total_bd_count_&_duration_2.vi"("Refnum in"=w15697, "BREAKDOWN_STK_HOLD_ID"=1, "condition"=w15688, "Form Date"=w15692, "To Date"=w15691, "error in (no error)"=w15695, "Shift"=w15687) -> ("Refnum out"=w15696:T2, "Count out"=w15690:string[], "appended array"=w15689:dbl[], "error out"=w15694:errorcluster)  [unwired: 5 in]
                          }
                          frame Enabled {
                          }
                        }
                        n2847 = call "NUMERIC TO STRING.vi"("appended array"=w15676) -> ("Array"=w15675:string[])  [unwired: 4 in]
                        n2848 = call "Insert_empty_element_with_zero.vi"("searched date"=w15679, "fixed date"=w15677) -> ("O/P"=w15672:string[])  [unwired: 9 in]
                        n2849 = call "Insert_empty_element_with_zero.vi"("searched date"=w15675, "fixed date"=w15677) -> ("O/P"=w15678:string[])  [unwired: 9 in]
                      }
                      frame #2 {
                        n2850 = disable-structure shown="Enabled" {
                          disable-tunnel: w15716 -> [w15730 w15732]
                          disable-tunnel: [w15729 w15732] -> w15715
                          disable-tunnel: w15714 -> [w15728 w15733]
                          disable-tunnel: [w15727 w15733] -> w15713
                          disable-tunnel: w15712 -> [w15726 _]
                          disable-tunnel: w15711 -> [w15725 _]
                          disable-tunnel: [w15724 _] -> w15710
                          disable-tunnel: [w15723 _] -> w15706
                          disable-tunnel: w15704 -> [w15722 _]
                          disable-tunnel: w15702 -> [w15720 w15731]
                          disable-tunnel: [_ w15731] -> w15701
                          frame Disabled {
                            n2851 = call "Stack_holderwise_total_bd_count_&_duration_2.vi"("Refnum in"=w15728, "BREAKDOWN_STK_HOLD_ID"=2, "condition"=w15722, "Form Date"=w15726, "To Date"=w15725, "error in (no error)"=w15730, "Shift"=w15720) -> ("Refnum out"=w15727:T2, "Count out"=w15724:string[], "appended array"=w15723:dbl[], "error out"=w15729:errorcluster)  [unwired: 5 in]
                          }
                          frame Enabled {
                          }
                        }
                        n2852 = call "Insert_empty_element_with_zero.vi"("searched date"=w15710, "fixed date"=w15707) -> ("O/P"=w15709:string[])  [unwired: 9 in]
                        n2853 = call "NUMERIC TO STRING.vi"("appended array"=w15706) -> ("Array"=w15705:string[])  [unwired: 4 in]
                        n2854 = call "Insert_empty_element_with_zero.vi"("searched date"=w15705, "fixed date"=w15707) -> ("O/P"=w15708:string[])  [unwired: 9 in]
                      }
                      frame #3 {
                        n2855 = disable-structure shown="Enabled" {
                          disable-tunnel: w15749 -> [w15765 w15767]
                          disable-tunnel: [w15764 w15767] -> w15748
                          disable-tunnel: w15747 -> [w15763 w15768]
                          disable-tunnel: [w15762 w15768] -> w15746
                          disable-tunnel: w15745 -> [w15761 _]
                          disable-tunnel: w15744 -> [w15760 _]
                          disable-tunnel: [w15759 _] -> w15743
                          disable-tunnel: [w15758 _] -> w15739
                          disable-tunnel: w15737 -> [w15757 _]
                          disable-tunnel: w15735 -> [w15755 w15766]
                          disable-tunnel: [_ w15766] -> w15734
                          frame Disabled {
                            n2856 = call "Stack_holderwise_total_bd_count_&_duration_2.vi"("Refnum in"=w15763, "BREAKDOWN_STK_HOLD_ID"=3, "condition"=w15757, "Form Date"=w15761, "To Date"=w15760, "error in (no error)"=w15765, "Shift"=w15755) -> ("Refnum out"=w15762:T2, "Count out"=w15759:string[], "appended array"=w15758:dbl[], "error out"=w15764:errorcluster)  [unwired: 5 in]
                          }
                          frame Enabled {
                          }
                        }
                        n2857 = call "Insert_empty_element_with_zero.vi"("searched date"=w15743, "fixed date"=w15740) -> ("O/P"=w15742:string[])  [unwired: 9 in]
                        n2858 = call "NUMERIC TO STRING.vi"("appended array"=w15739) -> ("Array"=w15738:string[])  [unwired: 4 in]
                        n2859 = call "Insert_empty_element_with_zero.vi"("searched date"=w15738, "fixed date"=w15740) -> ("O/P"=w15741:string[])  [unwired: 9 in]
                      }
                      frame #4 {
                        n2860 = call "Stack_holderwise_total_bd_count_&_duration_2.vi"("Refnum in"=w15783, "BREAKDOWN_STK_HOLD_ID"=4, "condition"=w15772, "Form Date"=w15780, "To Date"=w15779, "error in (no error)"=w15784, "Shift"=w15769) -> ("Refnum out"=w15782:T2, "Count out"=w15778:string[], "appended array"=w15774:dbl[], "error out"=w15781:errorcluster)  [unwired: 5 in]
                        n2861 = call "Insert_empty_element_with_zero.vi"("searched date"=w15778, "fixed date"=w15775) -> ("O/P"=w15777:string[])  [unwired: 9 in]
                        n2862 = call "NUMERIC TO STRING.vi"("appended array"=w15774) -> ("Array"=w15773:string[])  [unwired: 4 in]
                        n2863 = call "Insert_empty_element_with_zero.vi"("searched date"=w15773, "fixed date"=w15775) -> ("O/P"=w15776:string[])  [unwired: 9 in]
                      }
                      frame #5 {
                        n2864 = disable-structure shown="Enabled" {
                          disable-tunnel: w15805 -> [w15823 w15826]
                          disable-tunnel: [w15822 w15826] -> w15804
                          disable-tunnel: w15803 -> [w15821 w15825]
                          disable-tunnel: [w15820 w15825] -> w15802
                          disable-tunnel: w15801 -> [w15819 _]
                          disable-tunnel: w15800 -> [w15818 _]
                          disable-tunnel: [w15817 _] -> w15799
                          disable-tunnel: [w15816 _] -> w15795
                          disable-tunnel: w15793 -> [w15815 _]
                          frame Disabled {
                            n2865 = call "Stack_holderwise_total_bd_count_&_duration.vi"("Refnum in"=w15821, "BREAKDOWN_STK_HOLD_ID"=5, "condition"=w15815, "Form Date"=w15818, "To Date"=w15819, "error in (no error)"=w15823) -> ("Refnum out"=w15820:T2, "Count out"=w15817:string[], "appended array"=w15816:dbl[], "error out"=w15822:errorcluster)  [unwired: 6 in]
                          }
                          frame Enabled {
                          }
                        }
                        n2866 = call "NUMERIC TO STRING.vi"("appended array"=w15795) -> ("Array"=w15794:string[])  [unwired: 4 in]
                        n2867 = call "Insert_empty_element_with_zero.vi"("searched date"=w15799, "fixed date"=w15797) -> ("O/P"=w15798:string[])  [unwired: 9 in]
                        n2868 = call "Insert_empty_element_with_zero.vi"("searched date"=w15794, "fixed date"=w15797) -> ("O/P"=w15796:string[])  [unwired: 9 in]
                      }
                      frame #6 {
                        n2869 = call "String to numeric.vi"("Array"=w15837) -> ("Array 2"=w15836:dbl[])  [unwired: 4 in]
                        n2870 = call "String to numeric.vi"("Array"=w15835) -> ("Array 2"=w15834:dbl[])  [unwired: 4 in]
                        n2871 = call "String to numeric.vi"("Array"=w15833) -> ("Array 2"=w15832:dbl[])  [unwired: 4 in]
                        n2872 = call "String to numeric.vi"("Array"=w15831) -> ("Array 2"=w15830:dbl[])  [unwired: 4 in]
                        n2873 = call "String to numeric.vi"("Array"=w15829) -> ("Array 2"=w15828:dbl[])  [unwired: 4 in]
                        n2874 = Decimal String To Number(string=w15842) -> (number=w15861:i32[])  [unwired: 2 in, 1 out]
                        n2875 = Decimal String To Number(string=w15843) -> (number=w15862:i32[])  [unwired: 2 in, 1 out]
                        n2876 = Decimal String To Number(string=w15844) -> (number=w15863:i32[])  [unwired: 2 in, 1 out]
                        n2877 = Decimal String To Number(string=w15845) -> (number=w15864:i32[])  [unwired: 2 in, 1 out]
                        n2878 = Decimal String To Number(string=w15846) -> (number=w15859:i32[])  [unwired: 2 in, 1 out]
                        n2879 = Compound Arithmetic op=ADD(w15836, w15834, w15832, w15830, w15828) -> (w15839:dbl[])
                        n2880 = Build Array(w15837) -> (w15858:string[][])
                        n2881 = Build Array(w15835) -> (w15857:string[][])
                        n2882 = Build Array(w15833) -> (w15856:string[][])
                        n2883 = Build Array(w15831) -> (w15855:string[][])
                        n2884 = Build Array(w15829) -> (w15854:string[][])
                        n2885 = Number To Fractional String(number=w15839, precision (6)=i16 2) -> (F-format string=w15838:string[])  [unwired: 2 in]
                        n2886 = Compound Arithmetic op=ADD(w15861, w15862, w15863, w15864, w15859) -> (w15865:i32[])
                        n2887 = Transpose 2D Array(2D array=w15858) -> (transposed array=w15852:string[][])
                        n2888 = Transpose 2D Array(2D array=w15857) -> (transposed array=w15851:string[][])
                        n2889 = Transpose 2D Array(2D array=w15856) -> (transposed array=w15850:string[][])
                        n2890 = Transpose 2D Array(2D array=w15855) -> (transposed array=w15849:string[][])
                        n2891 = Transpose 2D Array(2D array=w15854) -> (transposed array=w15848:string[][])
                        n2892 = Number To Decimal String(number=w15865) -> (decimal integer string=w15860:string[])  [unwired: 1 in]
                        n2893 = Build Array(w15838) -> (w15841:string[][])
                        n2894 = Transpose 2D Array(2D array=w15841) -> (transposed array=w15847:string[][])
                      }
                      frame #7 {
                        w15870 = string[] [""]
                        n2895 = Insert Into Array(array=w15878, index (col)=1 ("disabled index (col)"), new element #1=w15870, new element #2=w15870, new element #3=w15870, new element #4=w15870, new element #5=w15870, new element #6=w15870, new element #7=w15869, new element #8=w15868, new element #9=w15870, new element #10=w15870, new element #11=w15871, new element #12=w15872) -> (w15874:string[][])  [unwired: 1 in]
                        n2896 = call "flot graph for month n year.vi"("BD Date"=w15875, "error in (no error)"=w15877, "Count total"=w15871) -> ("error out"=w15876:errorcluster, "Run-Time Status"=w15873:cluster{"Array 2":timestamp[], dbl[]})  [unwired: 7 in]
                        n2897 = local write "Run-Time Status"(w15873) -> ()
                        n2898 = local write "Table"(w15874) -> ()
                      }
                    }
                  }
                  frame "2" {
                    n2899 = flat-sequence {
                      tunnel: w15890 -> [w16004]
                      tunnel: w15889 -> [w16002]
                      tunnel: [w15988] -> w15980
                      tunnel: [w16003] -> w15979
                      tunnel: w15888 -> [_]
                      tunnel: [w16007] -> w15978
                      tunnel: [w15987] -> w15977
                      tunnel: [w15986] -> w15976
                      tunnel: [w15985] -> w15975
                      tunnel: w15887 -> [w15987]
                      tunnel: w15886 -> [w15986]
                      tunnel: ["Where BREAKDOWN_DATE between '%s'and '%s' and BREAKDOWN_STK_HOLD_ID ='%d' and  SHIFT_ID = '%d' "] -> w15974
                      tunnel: [w15985] -> w15973
                      tunnel: w15885 -> [w15981]
                      tunnel: [w15981] -> w15884
                      tunnel: w15980 -> [w16068]
                      tunnel: w15979 -> [w16070]
                      tunnel: w15978 -> [w16066]
                      tunnel: w15977 -> [w16065]
                      tunnel: w15976 -> [w16064]
                      tunnel: [w16067] -> w15972
                      tunnel: [w16069] -> w15971
                      tunnel: [w16066] -> w15970
                      tunnel: [w16056] -> w15969
                      tunnel: [w16062] -> w15968
                      tunnel: [w16065] -> w15967
                      tunnel: [w16064] -> w15966
                      tunnel: w15975 -> [w16061]
                      tunnel: [w16061] -> w15965
                      tunnel: w15974 -> [w16058]
                      tunnel: [w16058] -> w15964
                      tunnel: [w16057] -> w15963
                      tunnel: w15973 -> [w16057]
                      tunnel: w15884 -> [w16055]
                      tunnel: [w16054] -> w15883
                      tunnel: w15972 -> [w16100]
                      tunnel: w15971 -> [w16098]
                      tunnel: w15970 -> [w16103]
                      tunnel: w15969 -> [w16102]
                      tunnel: w15968 -> [w16101]
                      tunnel: w15967 -> [w16096]
                      tunnel: w15966 -> [w16095]
                      tunnel: [w16103] -> w15962
                      tunnel: [w16102] -> w15961
                      tunnel: [w16101] -> w15960
                      tunnel: [w16099] -> w15959
                      tunnel: [w16093] -> w15958
                      tunnel: [w16092] -> w15957
                      tunnel: [w16097] -> w15956
                      tunnel: [w16096] -> w15955
                      tunnel: [w16095] -> w15954
                      tunnel: w15965 -> [w16091]
                      tunnel: [w16091] -> w15953
                      tunnel: w15964 -> [w16088]
                      tunnel: [w16088] -> w15952
                      tunnel: [w16087] -> w15951
                      tunnel: w15963 -> [w16087]
                      tunnel: w15883 -> [w16086]
                      tunnel: [w16085] -> w15882
                      tunnel: w15962 -> [w16138]
                      tunnel: w15961 -> [w16137]
                      tunnel: w15960 -> [w16136]
                      tunnel: w15959 -> [w16133]
                      tunnel: w15958 -> [w16135]
                      tunnel: w15957 -> [w16134]
                      tunnel: w15956 -> [w16131]
                      tunnel: w15955 -> [w16129]
                      tunnel: w15954 -> [w16128]
                      tunnel: [w16138] -> w15950
                      tunnel: [w16137] -> w15949
                      tunnel: [w16136] -> w15948
                      tunnel: [w16135] -> w15947
                      tunnel: [w16134] -> w15946
                      tunnel: [w16132] -> w15945
                      tunnel: [w16126] -> w15944
                      tunnel: [w16125] -> w15943
                      tunnel: [w16130] -> w15942
                      tunnel: [w16129] -> w15941
                      tunnel: [w16128] -> w15940
                      tunnel: w15953 -> [w16124]
                      tunnel: [w16124] -> w15939
                      tunnel: w15952 -> [w16121]
                      tunnel: [w16121] -> w15938
                      tunnel: [w16120] -> w15937
                      tunnel: w15951 -> [w16120]
                      tunnel: w15882 -> [w16119]
                      tunnel: [w16118] -> w15881
                      tunnel: w15950 -> [w16175]
                      tunnel: w15949 -> [w16174]
                      tunnel: w15948 -> [w16173]
                      tunnel: w15947 -> [w16172]
                      tunnel: w15946 -> [w16171]
                      tunnel: w15945 -> [w16168]
                      tunnel: w15944 -> [w16170]
                      tunnel: w15943 -> [w16169]
                      tunnel: w15942 -> [w16167]
                      tunnel: w15941 -> [w16164]
                      tunnel: w15940 -> [w16163]
                      tunnel: [w16175] -> w15936
                      tunnel: [w16174] -> w15935
                      tunnel: [w16173] -> w15934
                      tunnel: [w16172] -> w15933
                      tunnel: [w16171] -> w15932
                      tunnel: [w16170] -> w15931
                      tunnel: [w16169] -> w15930
                      tunnel: [w16166] -> w15929
                      tunnel: [w16165] -> w15928
                      tunnel: [w16161] -> w15927
                      tunnel: [w16160] -> w15926
                      tunnel: [w16164] -> w15925
                      tunnel: [w16163] -> w15924
                      tunnel: w15939 -> [w16159]
                      tunnel: [w16159] -> w15923
                      tunnel: w15938 -> [w16156]
                      tunnel: [w16156] -> w15922
                      tunnel: [w16155] -> w15921
                      tunnel: w15937 -> [w16155]
                      tunnel: w15881 -> [w16153]
                      tunnel: w15936 -> [w16198]
                      tunnel: w15935 -> [w16197]
                      tunnel: w15934 -> [w16196]
                      tunnel: w15933 -> [w16195]
                      tunnel: w15932 -> [w16194]
                      tunnel: w15931 -> [w16193]
                      tunnel: w15930 -> [w16192]
                      tunnel: w15929 -> [w16187]
                      tunnel: w15928 -> [w16189]
                      tunnel: w15927 -> [w16191]
                      tunnel: w15926 -> [w16190]
                      tunnel: w15925 -> [w16184]
                      tunnel: w15924 -> [w16185]
                      tunnel: [w16198] -> w15920
                      tunnel: [w16197] -> w15919
                      tunnel: [w16196] -> w15918
                      tunnel: [w16195] -> w15917
                      tunnel: [w16194] -> w15916
                      tunnel: [w16193] -> w15915
                      tunnel: [w16192] -> w15914
                      tunnel: [w16191] -> w15913
                      tunnel: [w16190] -> w15912
                      tunnel: [w16188] -> w15911
                      tunnel: [w16186] -> w15910
                      tunnel: [w16182] -> w15909
                      tunnel: [w16180] -> w15908
